vi "Verify Timer.vi"(8 "error in (no error)":errorcluster, 11 "State Machine in":refnum<class "CM_State Machine.lvclass">) -> (0 "error out":errorcluster, 2 "time out":bool, 3 "State Machine out":refnum<class "CM_State Machine.lvclass">)   [LabVIEW 2018, in "CM_State Machine.lvclass"]
doc: "Verify the time of the class"
uses:
  CM_State Machine.lvclass
  CM_State Machine.lvclass/CM_State Machine.ctl
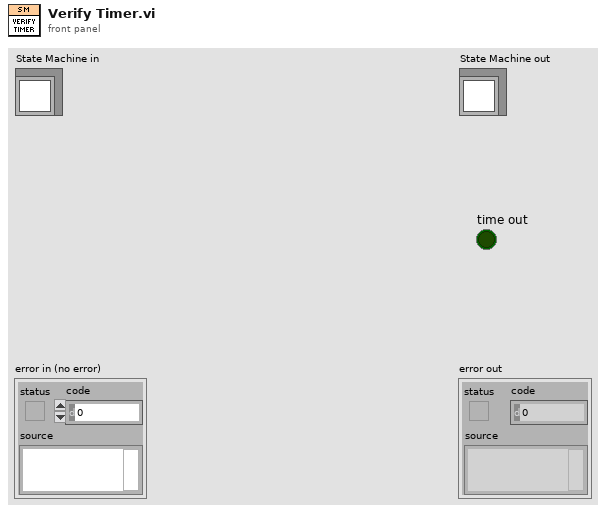
[diagram p1: front panel]
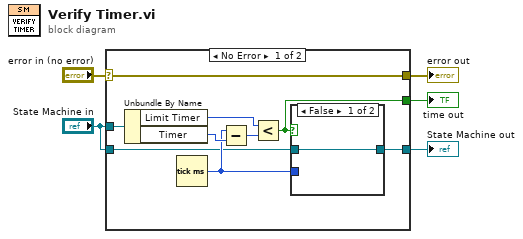
[diagram p0: block diagram]
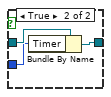
[diagram p2: hidden frame]
diagram:
  n1 = case shown="No Error" "error in (no error)" {
    selector: "error in (no error)" -> [w14 w20]
    tunnel: [w14 w20] -> w4
    tunnel: [w7 w19] -> w3
    tunnel: "State Machine in" -> [w9 w19]
    tunnel: "State Machine in" -> [w8 _]
    tunnel: [w6 _] -> w1
    frame No Error {
      n2 = Unbundle By Name(w9) -> ("Limit Timer"=w11:u32, "Timer"=w13:u32)
      n3 = Tick Count (ms)() -> (millisecond timer value=w10:u32)
      n4 = Subtract(x=w10, y=w13) -> (x-y=w12:u32)
      n5 = Less?(x=w11, y=w12) -> (x < y?=w6:bool)
      n6 = case shown="False" w6 {
        tunnel: w10 -> [_ w16]
        tunnel: w8 -> [w15 w18]
        tunnel: [w15 w17] -> w7
        frame False {
        }
        frame True {
          n7 = Bundle By Name(cluster=w18, "Timer"=w16) -> (w17:refnum<class "CM_State Machine.lvclass">)
        }
      }
    }
    frame Error {
    }
  }
  "error out" <- w4
  "State Machine out" <- w3
  "time out" <- w1
